vi "Migrate Common Dependencies.vi"(0 "Project path":path, 5 "Measurement path":path, 7 "Dependencies path":path[](array[path]), 11 "error in (no error)":errorcluster) -> (4 "Project reference":refnum<vi>, 6 "MeasurementCore reference":refnum<vi>, 8 "Outside items":string[](array[string]), 10 "Library":T1[](array[typedef]), 15 "error out":errorcluster)   [LabVIEW 2021, in "Multiple Migrator.lvlib"]
uses:
  Multiple Migrator.lvlib
  controls/Library Info.ctl
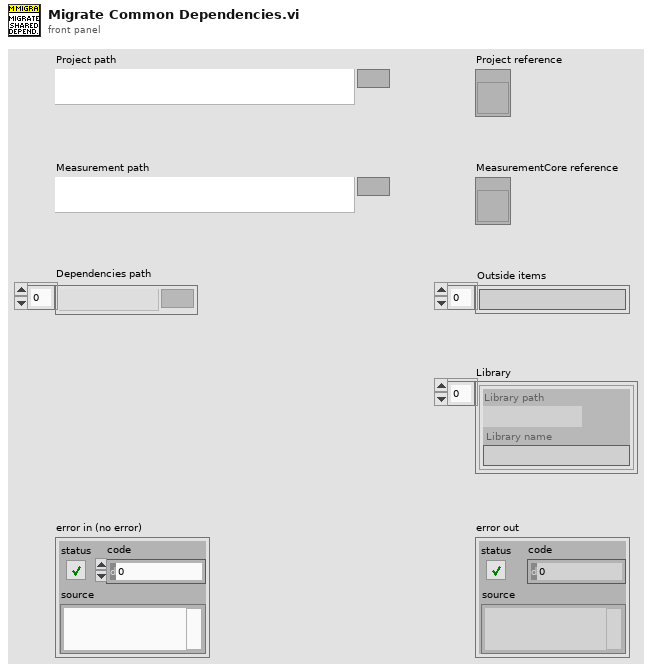
[diagram p1: front panel]
types:
  T1 = typedef "Multiple Migrator.lvlib/Library Info.ctl" = cluster{"Library path":path, "Library name":string}
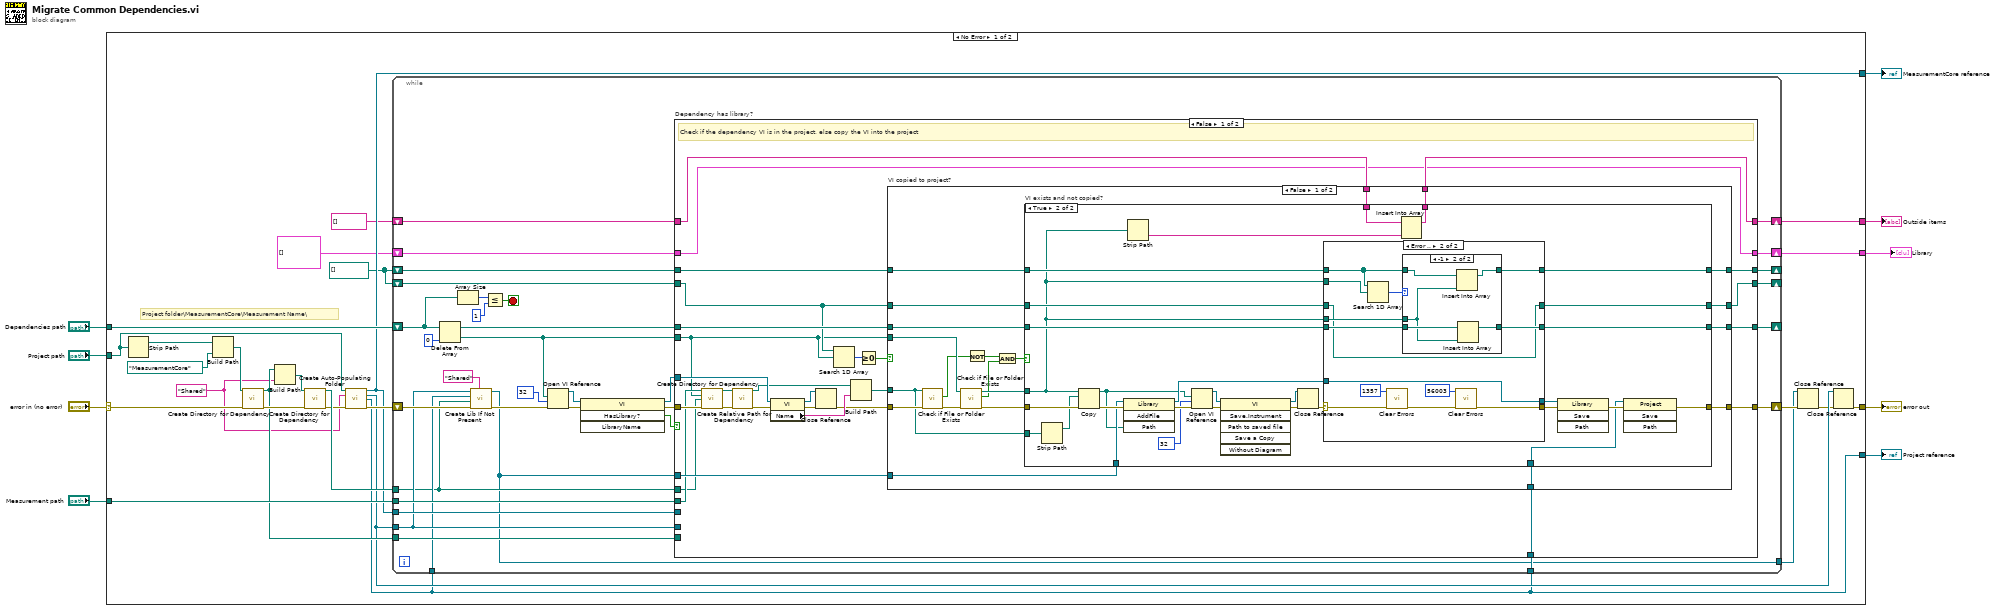
[diagram p0: block diagram]
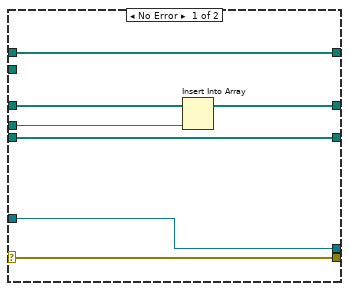
[diagram p3: hidden frame]
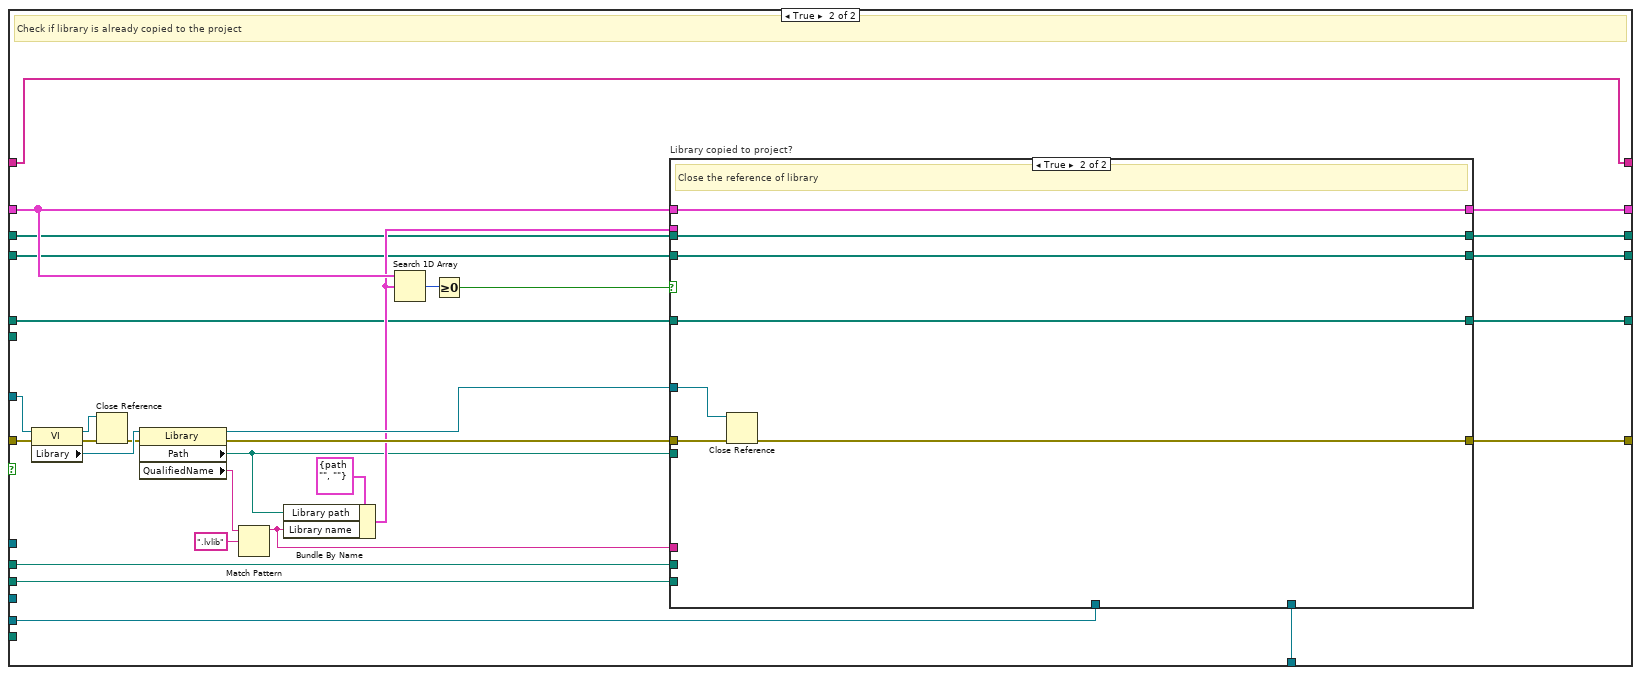
[diagram p6: hidden frame]
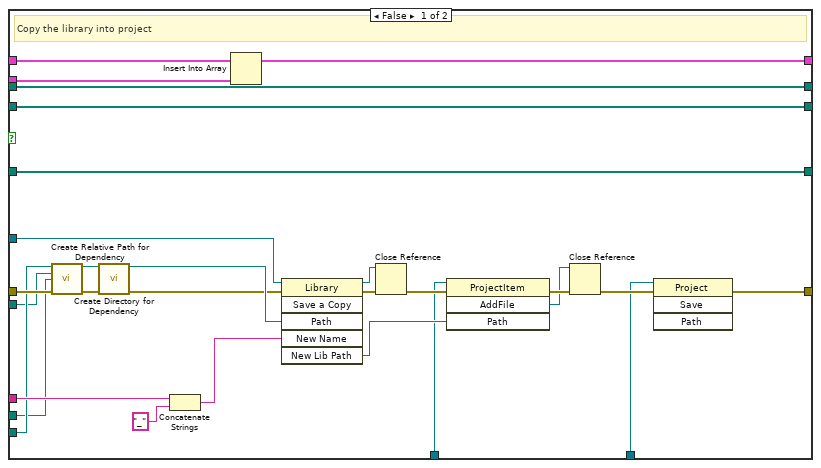
[diagram p7: hidden frame]
diagram:
  n1 = case shown="No Error" "error in (no error)" {
    selector: "error in (no error)" -> [w27 w251]
    tunnel: [w20 w251] -> w8
    tunnel: "Project path" -> [w26 _]
    tunnel: "Measurement path" -> [w31 _]
    tunnel: "Dependencies path" -> [w35 _]
    tunnel: [w22 _] -> w4
    tunnel: [w16 _] -> w3
    tunnel: [w17 _] -> w2
    tunnel: [w10 _] -> w1
    frame No Error {
      w12 = "Shared"
      w13 = path[] []
      # "Project folder\\MeasurementCore\\Measurement Name\\"
      n2 = Strip Path(path=w26) -> (stripped path=w30:path)  [unwired: 1 out]
      n3 = Build Path(base path=w30, name or relative path=path "MeasurementCore") -> (appended path=w28:path)
      n4 = call "Create Directory for Dependency.vi"("Directory path"=w28, "error in (no error)"=w27) -> ("Directory path out"=w21:path, "error out"=w25:errorcluster)  [unwired: 12 in]
      n5 = Build Path(base path=w21, name or relative path=w12) -> (appended path=w34:path)
      n6 = call "Create Directory for Dependency.vi"("Directory path"=w34, "error in (no error)"=w25) -> ("Directory path out"=w33:path, "error out"=w24:errorcluster)  [unwired: 12 in]
      n7 = call "Create Auto-Populating Folder.vi"("Project path"=w26, "Plug-in name"=w12, "error in (no error)"=w24) -> ("MeasurementCore reference"=w22:refnum<vi>, "Folder reference"=w19:refnum<vi>, "Project reference"=w16:refnum<vi>, "error out"=w23:errorcluster)  [unwired: 9 in]
      n8 = while {
        shift-right: [w57] -> w32
        shift-left: w23 -> [w45]
        shift-right: [w50] -> _
        shift-left: w35 -> [w67]
        tunnel: w33 -> [w41]
        shift-right: [w56] -> w10
        shift-left: T1[] [] -> [w59]
        tunnel: w31 -> [w55]
        shift-right: [w52] -> _
        shift-left: w13 -> [w53]
        tunnel: w22 -> [w49]
        tunnel: w21 -> [w48]
        tunnel: w19 -> [w43]
        shift-right: [w46] -> w17
        shift-left: string[] [] -> [w47]
        tunnel: w16 -> [w42]
        tunnel: w16 -> [w40]
        shift-right: [w39] -> _
        shift-left: w13 -> [w38]
        tunnel: [w37] -> w14
        stop <- w66 stop-if-true
        n9 = Delete From Array(array=w67, index=0) -> (deleted portion=w54:path, array with subset deleted=w51:path[])  [unwired: 1 in]
        n10 = Array Size(array=w67) -> (size(s)=w69:i32)
        n11 = call "Create Lib If Not Present.vi"("Plug-in name"="Shared", "error in (no error)"=w45, "DestDirectory"=w41, "ProjectRef"=w42, "VirtualFolderRef"=w43) -> ("error out"=w44:errorcluster, "Library Refnum"=w37:refnum<vi>)  [unwired: 5 in]
        n12 = Less Or Equal?(x=w69, y=1) -> (x <= y?=w66:bool)
        n13 = Open VI Reference(vi path=w54, options=32, error in (no error)=w44) -> (vi reference=w63:refnum<vi>, error out=w65:errorcluster)  [unwired: 3 in]
        n14 = invoke class="VI" method="HasLibrary?"(reference=w63, error in=w65) -> (reference out=w60:refnum<vi>, error out=w61:errorcluster, "Has Library?"=w62:bool)  [unwired: 2 in, 1 out]
        n15 = case "Dependency has library?" shown="False" w62 {
          tunnel: w61 -> [w75 w214]
          tunnel: w60 -> [w96 w215]
          tunnel: w59 -> [w79 w202]
          tunnel: [w91 w203] -> w57
          tunnel: [w79 w201] -> w56
          tunnel: w55 -> [w74 w199]
          tunnel: w41 -> [w72 w197]
          tunnel: w54 -> [w73 _]
          tunnel: w53 -> [w87 w194]
          tunnel: [w83 w193] -> w52
          tunnel: w51 -> [w90 w192]
          tunnel: [w89 w191] -> w50
          tunnel: w49 -> [_ _]
          tunnel: w48 -> [_ _]
          tunnel: w43 -> [_ w190]
          tunnel: w47 -> [w81 w189]
          tunnel: [w80 w189] -> w46
          tunnel: w37 -> [w82 _]
          tunnel: w40 -> [w76 w188]
          tunnel: [w78 w186] -> w39
          tunnel: w38 -> [w77 w187]
          frame False {
            # "Check if the dependency VI is in the project, else copy the VI into the project"
            n16 = call "Create Relative Path for Dependency.vi"("Old Main Path"=w74, "Old Dependency Path"=w73, "New Dir"=w72, "error in (no error)"=w75) -> ("Directory"=w70:path, "error out"=w71:errorcluster)  [unwired: 10 in]
            n17 = call "Create Directory for Dependency.vi"("Directory path"=w70, "error in (no error)"=w71) -> ("Directory path out"=w88:path, "error out"=w97:errorcluster)  [unwired: 12 in]
            n18 = property class="VI"(reference=w96, error in=w97) -> (reference out=w92:refnum<vi>, error out=w95:errorcluster, "Name"=w94:string)
            n19 = Close Reference(reference=w92, error in (no error)=w95) -> (error out=w93:errorcluster)
            n20 = Search 1D Array(1D array=w87, element=w73) -> (index of element=w86:i32)  [unwired: 1 in]
            n21 = Build Path(base path=w88, name or relative path=w94) -> (appended path=w85:path)
            n22 = Greater Or Equal To 0?(x=w86) -> (x >= 0?=w84:bool)
            n23 = case "VI copied to project?" shown="False" w84 {
              tunnel: w93 -> [w118 w185]
              tunnel: w73 -> [w117 _]
              tunnel: [w114 w185] -> w91
              tunnel: w87 -> [w113 w184]
              tunnel: [w112 w184] -> w83
              tunnel: w85 -> [w108 _]
              tunnel: w90 -> [w111 w183]
              tunnel: [w110 w183] -> w89
              tunnel: w81 -> [w103 w182]
              tunnel: [w102 w182] -> w80
              tunnel: w82 -> [w101 _]
              tunnel: [w100 w181] -> w78
              tunnel: w77 -> [w99 w181]
              tunnel: w76 -> [w98 _]
              frame False {
                n24 = call <vilib>:"Check if File or Folder Exists.vi"("error in (no error)"=w118, "path"=w108) -> ("error out"=w109:errorcluster, "file or folder exists?"=w107:bool)  [unwired: 7 in, 1 out]
                n25 = call <vilib>:"Check if File or Folder Exists.vi"("error in (no error)"=w109, "path"=w117) -> ("error out"=w116:errorcluster, "file or folder exists?"=w105:bool, "dup path"=w115:path)  [unwired: 7 in]
                n26 = Not(x=w107) -> (.not. x?=w106:bool)
                n27 = And(x=w106, y=w105) -> (x .and. y?=w104:bool)
                n28 = case "VI exists and not copied?" shown="True" w104 {
                  tunnel: w116 -> [w123 w152]
                  tunnel: w115 -> [_ w132]
                  tunnel: [w123 w134] -> w114
                  tunnel: w113 -> [w122 w151]
                  tunnel: [w122 w150] -> w112
                  tunnel: w108 -> [_ w146]
                  tunnel: w111 -> [w121 w136]
                  tunnel: [w121 w135] -> w110
                  tunnel: w103 -> [w120 w145]
                  tunnel: [w120 w143] -> w102
                  tunnel: w101 -> [_ w142]
                  tunnel: [w119 w141] -> w100
                  tunnel: w99 -> [w119 w140]
                  tunnel: w98 -> [_ w133]
                  frame False {
                  }
                  frame True {
                    n29 = Strip Path(path=w146) -> (stripped path=w148:path)  [unwired: 1 out]
                    n30 = Copy(8:w152, 10:w148, 11:w132) -> (0:w149:errorcluster, 3:w130:path)  [unwired: 2 in, 1 out]
                    n31 = invoke class="Library" method="AddFile"(reference=w142, error in=w149, "Path"=w130) -> (reference out=w139:refnum<vi>, error out=w131:errorcluster)  [unwired: 1 in, 2 out]
                    n32 = Strip Path(path=w132) -> (name=w144:string)  [unwired: 1 out]
                    n33 = Open VI Reference(vi path=w130, options=32, error in (no error)=w131) -> (vi reference=w128:refnum<vi>, error out=w124:errorcluster)  [unwired: 3 in]
                    n34 = invoke class="VI" method="Save.Instrument"(reference=w128, error in=w124) -> (reference out=w126:refnum<vi>, error out=w127:errorcluster)  [unwired: 4 in, 4 out]
                    n35 = Close Reference(reference=w126, error in (no error)=w127) -> (error out=w125:errorcluster)
                    n36 = case shown="Error .." w125 {
                      selector: w125 -> [w154 w173]
                      tunnel: w151 -> [w159 w160]
                      tunnel: [w158 w160] -> w150
                      tunnel: w132 -> [w157 w163]
                      tunnel: [w156 w164] -> w141
                      tunnel: w140 -> [w156 w165]
                      tunnel: [w155 w162] -> w137
                      tunnel: w139 -> [w155 w162]
                      tunnel: [w154 w171] -> w138
                      tunnel: w136 -> [w153 w167]
                      tunnel: [w153 w166] -> w135
                      tunnel: w132 -> [_ w168]
                      frame No Error {
                        n37 = Insert Into Array(array=w159, new element=w157) -> (w158:path[])  [unwired: 1 in]
                      }
                      frame Error {
                        n38 = Search 1D Array(1D array=w165, element=w168) -> (index of element=w161:i32)  [unwired: 1 in]
                        n39 = call <vilib>:"Clear Errors.vi"("error in (no error)"=w173, "specific error code to clear (0: all)"=1357) -> ("error out"=w172:errorcluster)  [unwired: 4 in, 1 out]
                        n40 = case shown="-1" w161 {
                          tunnel: w167 -> [w174 w180]
                          tunnel: [w174 w179] -> w166
                          tunnel: w165 -> [w175 w178]
                          tunnel: [w175 w177] -> w164
                          tunnel: w163 -> [_ w176]
                          frame Default {
                          }
                          frame -1 {
                            n41 = Insert Into Array(array=w178, new element=w176) -> (w177:path[])  [unwired: 1 in]
                            n42 = Insert Into Array(array=w180, new element=w176) -> (w179:path[])  [unwired: 1 in]
                          }
                        }
                        n43 = call <vilib>:"Clear Errors.vi"("error in (no error)"=w172, "specific error code to clear (0: all)"=56003) -> ("error out"=w171:errorcluster)  [unwired: 4 in, 1 out]
                      }
                    }
                    n44 = Insert Into Array(array=w145, new element=w144) -> (w143:string[])  [unwired: 1 in]
                    n45 = invoke class="Library" method="Save"(reference=w137, error in=w138) -> (error out=w147:errorcluster)  [unwired: 2 in, 3 out]
                    n46 = invoke class="Project" method="Save"(reference=w133, error in=w147) -> (error out=w134:errorcluster)  [unwired: 2 in, 3 out]
                  }
                }
              }
              frame True {
              }
            }
          }
          frame True {
            # "Check if library is already copied to the project"
            n47 = property class="VI"(reference=w215, error in=w214) -> (reference out=w205:refnum<vi>, error out=w213:errorcluster, "Library"=w212:refnum<vi>)
            n48 = Close Reference(reference=w205, error in (no error)=w213) -> (error out=w206:errorcluster)
            n49 = property class="Library"(reference=w212, error in=w206) -> (reference out=w204:refnum<vi>, error out=w207:errorcluster, "Path"=w198:path, "QualifiedName"=w208:string)
            n50 = Match Pattern(string=w208, regular expression=".lvlib") -> (before substring=w195:string)  [unwired: 1 in, 3 out]
            n51 = Bundle By Name(cluster=T1 {"Library path"=path "", "Library name"=""} ("Cluster"), "Library path"=w198, "Library name"=w195) -> (w200:T1)
            n52 = Search 1D Array(1D array=w202, element=w200) -> (index of element=w210:i32)  [unwired: 1 in]
            n53 = Greater Or Equal To 0?(x=w210) -> (x >= 0?=w209:bool)
            n54 = case "Library copied to project?" shown="True" w209 {
              tunnel: w207 -> [w220 w249]
              tunnel: w204 -> [w237 w250]
              tunnel: [w224 w248] -> w203
              tunnel: w202 -> [w243 w247]
              tunnel: [w242 w247] -> w201
              tunnel: w200 -> [w241 _]
              tunnel: w199 -> [w219 _]
              tunnel: w198 -> [w218 _]
              tunnel: w197 -> [w217 _]
              tunnel: w195 -> [w227 _]
              tunnel: w194 -> [w234 w246]
              tunnel: [w234 w246] -> w193
              tunnel: [w233 w245] -> w191
              tunnel: w192 -> [w233 w245]
              tunnel: w190 -> [w228 _]
              tunnel: w188 -> [w223 _]
              tunnel: [w222 w244] -> w186
              tunnel: w187 -> [w222 w244]
              frame False {
                # "Copy the library into project"
                n55 = call "Create Relative Path for Dependency.vi"("Old Main Path"=w219, "Old Dependency Path"=w218, "New Dir"=w217, "error in (no error)"=w220) -> ("Directory"=w216:path, "error out"=w221:errorcluster)  [unwired: 10 in]
                n56 = call "Create Directory for Dependency.vi"("Directory path"=w216, "error in (no error)"=w221) -> ("Directory path out"=w238:path, "error out"=w236:errorcluster)  [unwired: 12 in]
                n57 = Concatenate Strings(w227, "_" ("string")) -> (w225:string)
                n58 = Insert Into Array(array=w243, new element=w241) -> (w242:T1[])  [unwired: 1 in]
                n59 = invoke class="Library" method="Save a Copy"(reference=w237, error in=w236, "Path"=w238, "New Name"=w225) -> (reference out=w239:refnum<vi>, error out=w240:errorcluster, "New Lib Path"=w231:path)  [unwired: 2 in, 3 out]
                n60 = Close Reference(reference=w239, error in (no error)=w240) -> (error out=w235:errorcluster)
                n61 = invoke class="ProjectItem" method="AddFile"(reference=w228, error in=w235, "Path"=w231) -> (error out=w232:errorcluster, "AddFile"=w229:refnum<vi>)  [unwired: 1 in, 2 out]
                n62 = Close Reference(reference=w229, error in (no error)=w232) -> (error out=w230:errorcluster)
                n63 = invoke class="Project" method="Save"(reference=w223, error in=w230) -> (error out=w224:errorcluster)  [unwired: 2 in, 3 out]
              }
              frame True {
                # "Close the reference of library"
                n64 = Close Reference(reference=w250, error in (no error)=w249) -> (error out=w248:errorcluster)
              }
            }
          }
        }
      }
      n65 = Close Reference(reference=w14, error in (no error)=w32) -> (error out=w15:errorcluster)
      n66 = Close Reference(reference=w19, error in (no error)=w15) -> (error out=w20:errorcluster)
    }
    frame Error {
    }
  }
  "error out" <- w8
  "MeasurementCore reference" <- w4
  "Project reference" <- w3
  "Outside items" <- w2
  "Library" <- w1
